vi "Down Shift.vi"(8 "Error in":errorcluster) -> (0 "Error Out":errorcluster)   [LabVIEW 2014]
uses:
  <vilib>/Rock Robotics/WPI/Solenoid/WPI_SolenoidValue.ctl
  Global Objects.vi
  <vilib>/Rock Robotics/WPI/Solenoid/WPI_SolenoidSetEnum.vi
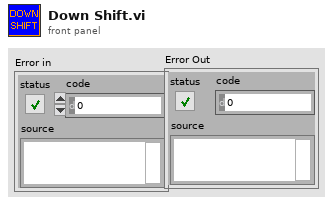
[diagram p1: front panel]
types:
  T1 = typedef "Shifter.ctl" = cluster{"SolenoidDevRef":T2}
  T2 = typedef "WPI_SolenoidDevRef.ctl" = cluster{"DevStatus":errorcluster, "Pneumatics Control Module":u8, "Forward Solenoid Channel":T3, "Reverse Solenoid Channel":T3}
  T3 = typedef "WPI_SolenoidChannel.ctl" = enum8{"Solenoid 0", "Solenoid 1", "Solenoid 2", "Solenoid 3", "Solenoid 4", "Solenoid 5", "Solenoid 6", "Solenoid 7", "Invalid"}
  T4 = typedef "WPI_SolenoidValue.ctl" = enum16{"Off", "On", "Forward", "Reverse"}
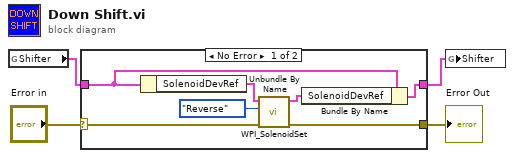
[diagram p0: block diagram]
diagram:
  n1 = global read "Global Objects.vi" "Shifter"() -> (w1:T1)
  n2 = case shown="No Error" "Error in" {
    selector: "Error in" -> [w9 w13]
    tunnel: [w8 w13] -> w3
    tunnel: [w5 w12] -> w2
    tunnel: w1 -> [w6 w12]
    frame No Error {
      n3 = Unbundle By Name(w6) -> ("SolenoidDevRef"=w11:T2)
      n4 = call-poly <vilib>:"WPI_SolenoidSet.vi"("error in (no error)"=w9, "Value"=WPI_SolenoidValue."Reverse", "SolenoidDevRef"=w11) -> ("error out"=w8:errorcluster, "SolenoidDevRef"=w7:T2)  [unwired: 7 in]
      n5 = Bundle By Name(cluster=w6, "SolenoidDevRef"=w7) -> (w5:T1)
    }
    frame Error {
    }
  }
  "Error Out" <- w3
  n6 = global write "Global Objects.vi" "Shifter"(w2) -> ()
